vi "Bin WebDav Logging Message Loop.vi"(8 "error in (no error)":errorcluster, 10 "Data Queue":refnum<queue>, 11 "Message Queues":T1) -> (0 "error out":errorcluster)   [LabVIEW 2018, in "Logging.lvlib"]
uses:
  Logging.lvlib
  support/Message Queue/All Message Queues.ctl
  support/Message Queue/Message Cluster.ctl
  Logging Configuration.ctl
  Logging State.ctl
  support/Message Queue/Enqueue Message (Single).vi
  <vilib>/Utility/error.llb/Error Cluster From Error Code.vi
  <vilib>/ErrorRing/Error Ring.xnode
  support/Message Queue/Message Queue.lvlib
  Acquisition/Acquisition.lvlib
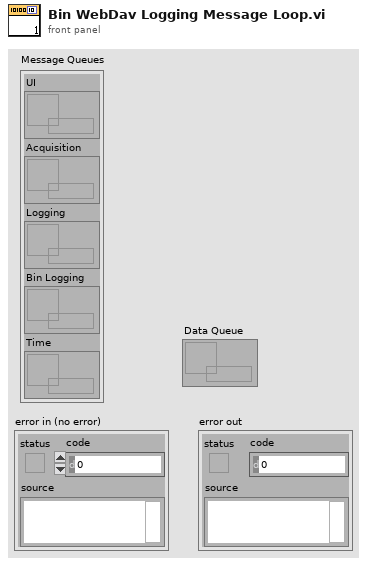
[diagram p1: front panel]
types:
  T1 = typedef "Message Queue.lvlib/All Message Queues.ctl" = cluster{"UI":refnum<queue>, "Acquisition":refnum<queue>, "Logging":refnum<queue>, "Bin Logging":refnum<queue>, "Time":refnum<queue>}
  T2 = typedef "Logging.lvlib/Logging Configuration.ctl" = cluster{"Log File Base Path":path, "TDMS File Reference":refnum<k34>, "Log File Offsite Path":path, "Project code":string, "Bin File Reference":refnum<k34>}
  T3 = typedef "Logging.lvlib/Logging State.ctl" = enum16{"Idle", "Logging"}
  T4 = enum16{"open", "open or create", "create or replace", "create", "open (read-only)"}
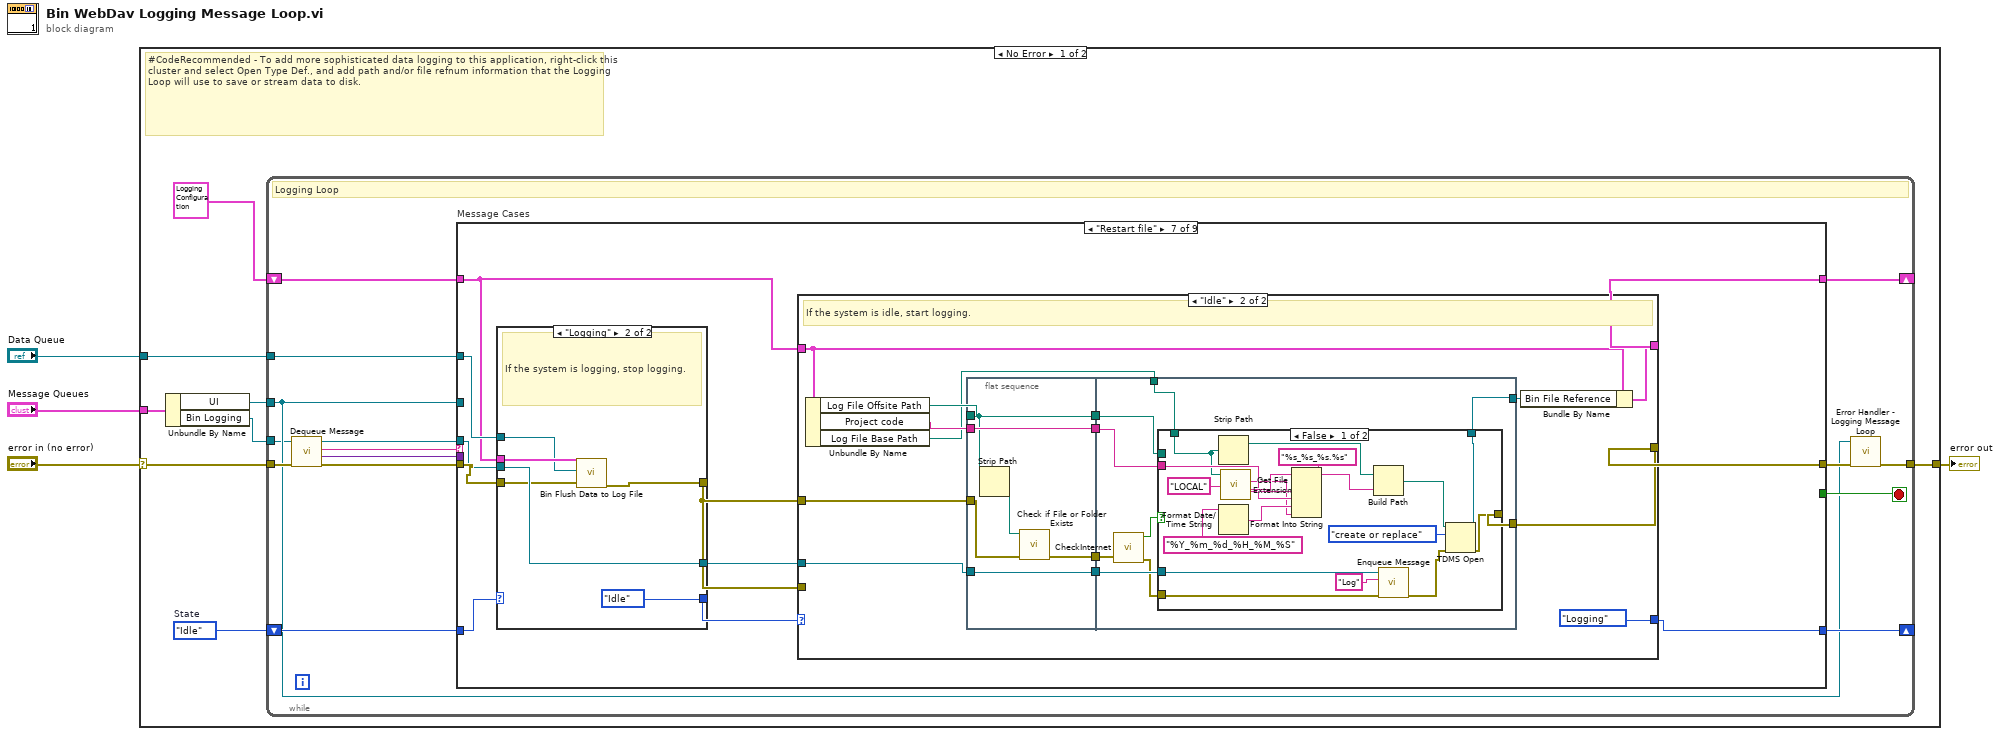
[diagram p0: block diagram]
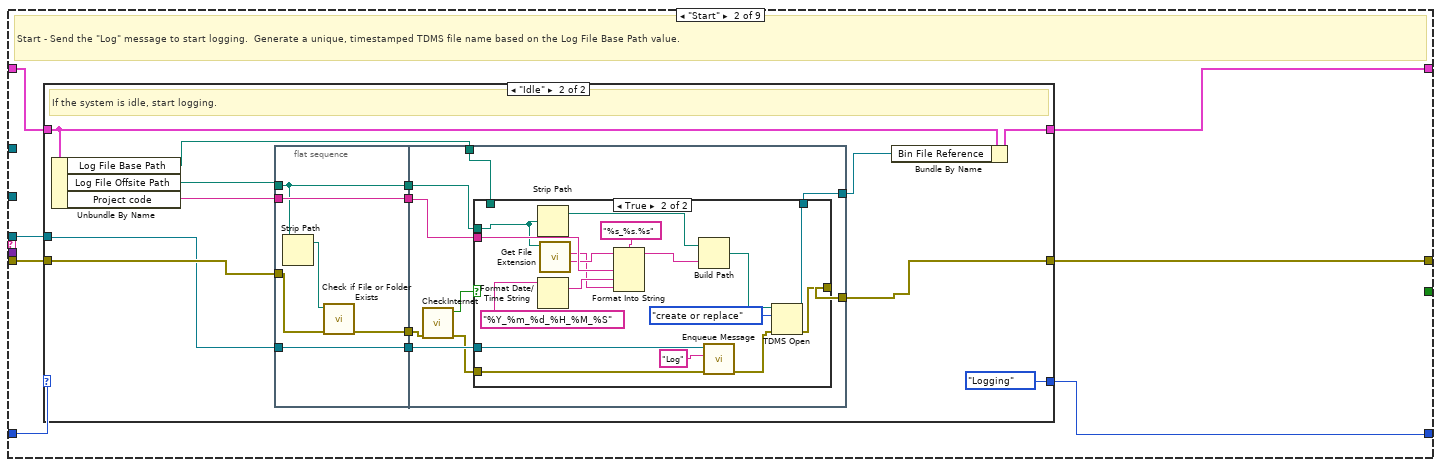
[diagram p3: hidden frame]
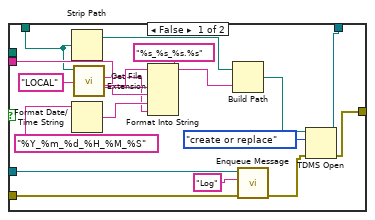
[diagram p5: hidden frame]
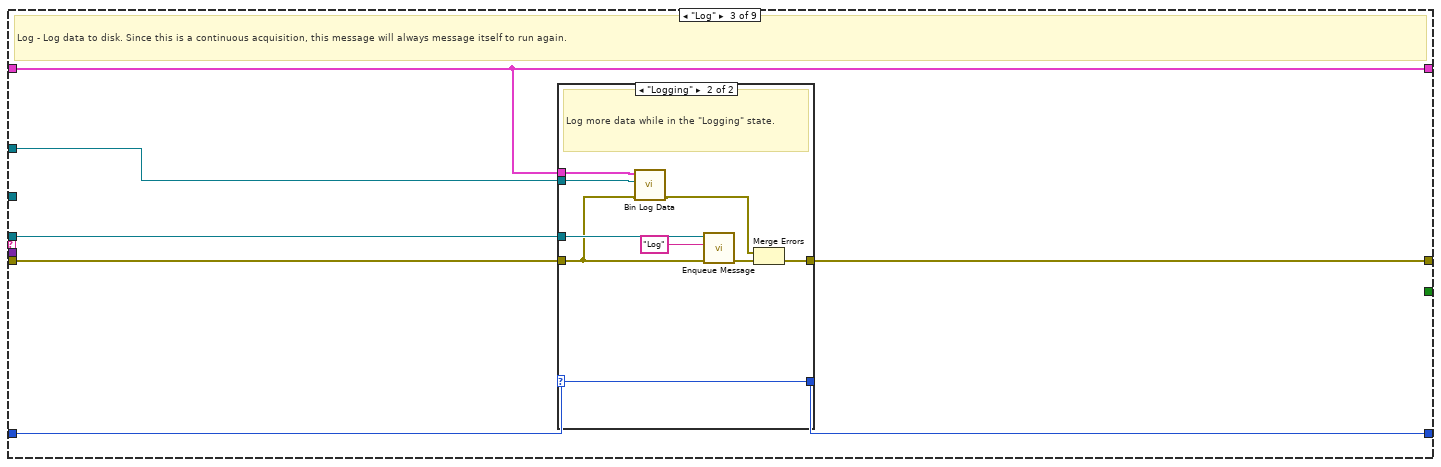
[diagram p6: hidden frame]
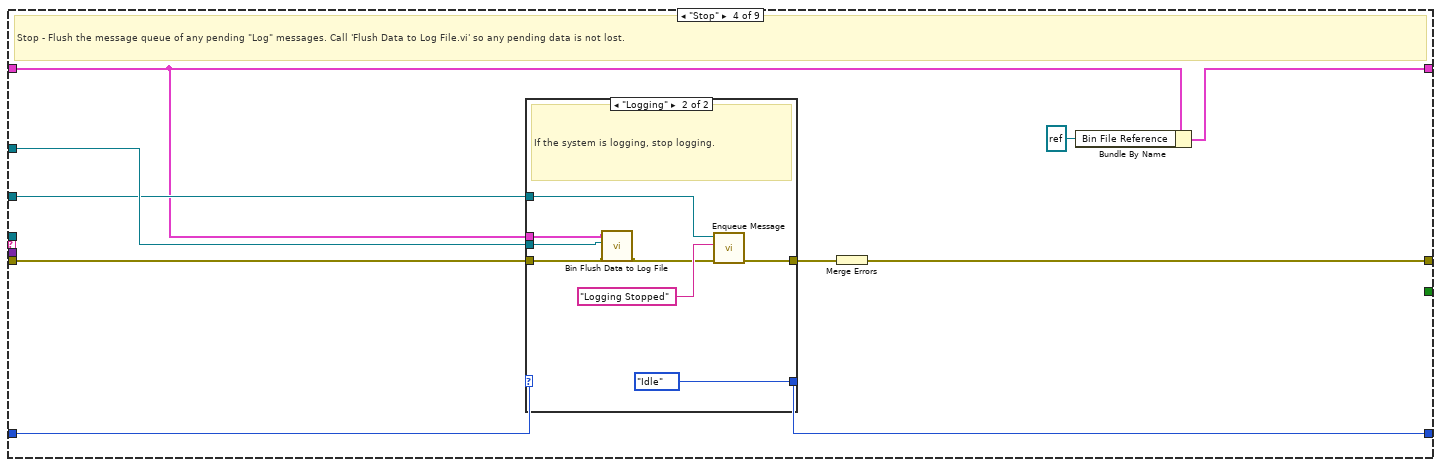
[diagram p8: hidden frame]
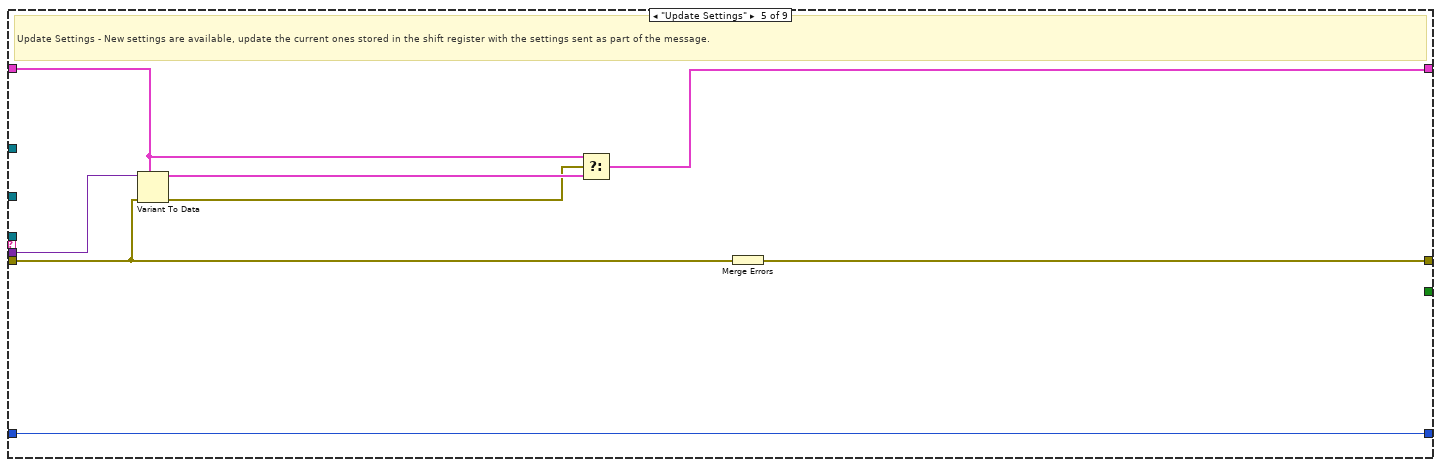
[diagram p10: hidden frame]
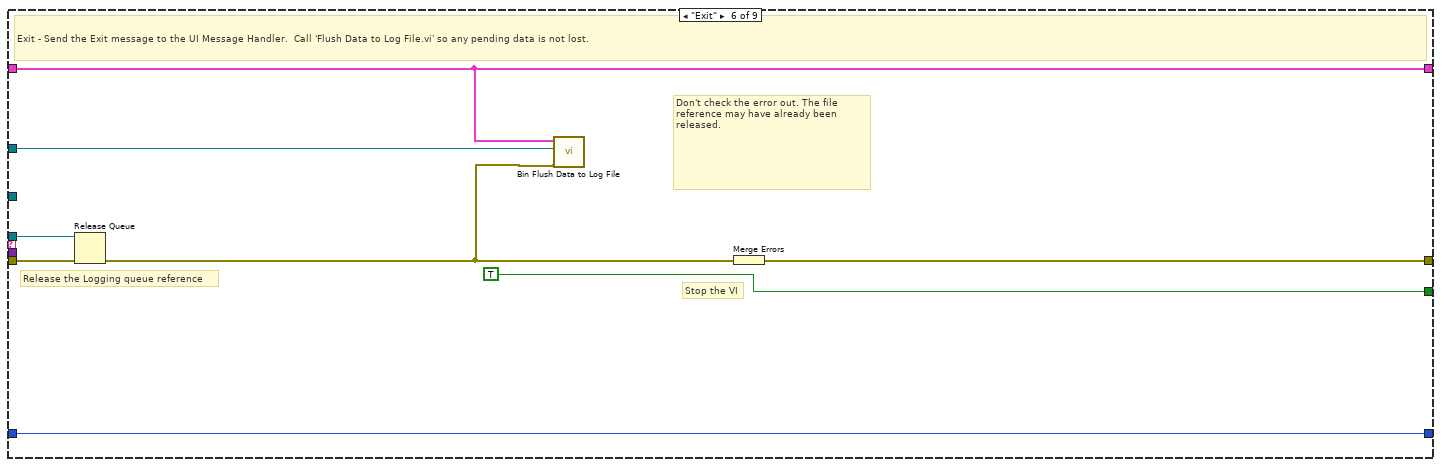
[diagram p11: hidden frame]
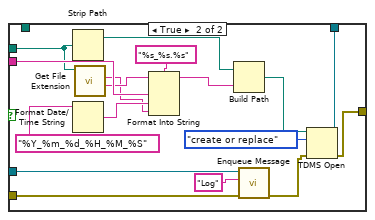
[diagram p13: hidden frame]
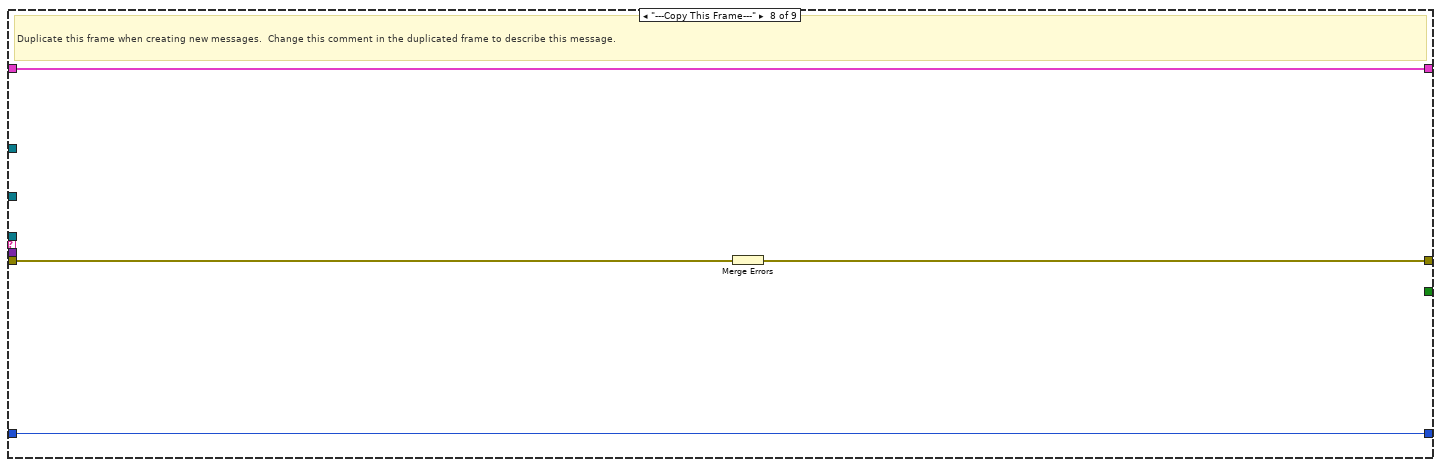
[diagram p15: hidden frame]
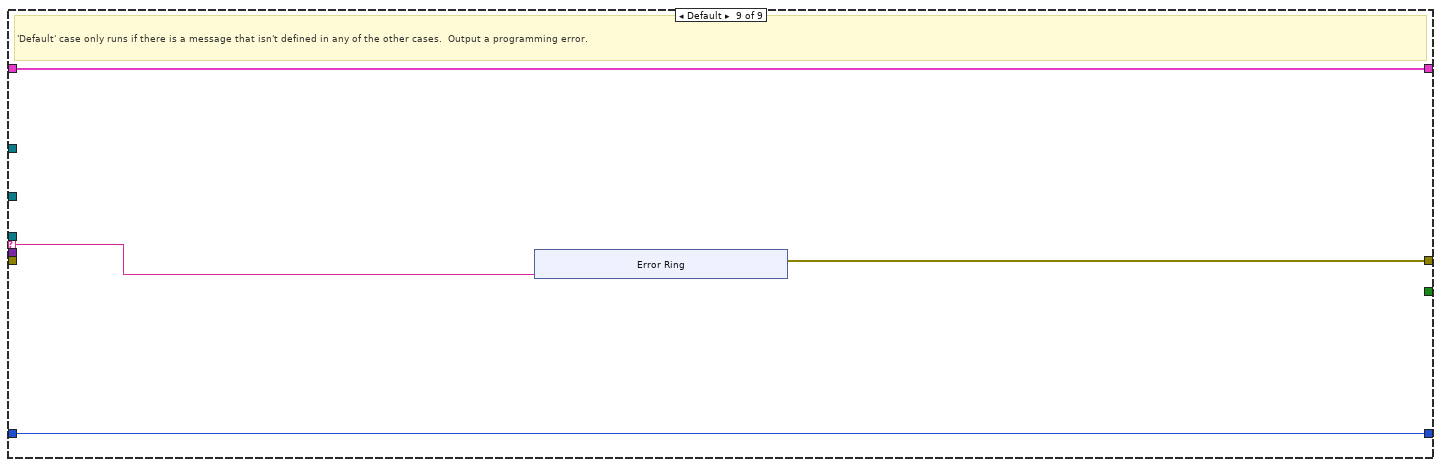
[diagram p16: hidden frame]
diagram:
  n1 = case shown="No Error" "error in (no error)" {
    selector: "error in (no error)" -> [w9 w256]
    tunnel: "Message Queues" -> [w12 _]
    tunnel: [w11 w256] -> w3
    tunnel: "Data Queue" -> [w8 _]
    frame No Error {
      w6 = Logging_State."Idle"  # State
      # "#CodeRecommended - To add more sophisticated data logging to this application, right-click this cluster and select Open Type Def., and add path and/or file refnum information that the Logging Loop will use to save or stream data to disk."
      n2 = Unbundle By Name(w12) -> ("UI"=w7:refnum<queue>, "Bin Logging"=w5:refnum<queue>)
      n3 = while {
        shift-right: [w27] -> _
        shift-left: T2 {"Log File Base Path"=path "", "TDMS File Reference"=refnum, "Log File Offsite Path"=path "", "Project code"="", "Bin File Reference"=refnum} ("Logging Configuration") -> [w14]
        tunnel: w7 -> [w16]
        tunnel: w8 -> [w21]
        shift-right: [w19] -> _
        shift-left: w6 -> [w20]
        tunnel: w9 -> [w25]
        tunnel: [w18] -> w11
        tunnel: w5 -> [w15]
        stop <- w26 stop-if-true
        # "Logging Loop"
        n4 = call "Dequeue Message.vi"("error in (no error)"=w25, "Message Queue"=w15) -> ("error out"=w24:errorcluster, "Message Data"=w23:variant, "Message"=w13:string, "dup Message Queue"=w22:refnum<queue>)  [unwired: 6 in]
        n5 = case "Message Cases" shown="\"Restart file\"" w13 {
          selector: w13 -> [_ _ _ _ _ _ _ _ w245]
          tunnel: w22 -> [_ w36 w108 _ _ w153 w166 _ _]
          tunnel: w24 -> [w29 w35 w106 w127 w141 w154 w167 w244 _]
          tunnel: [w29 w37 w109 w130 w148 w155 w165 w242 w246] -> w17
          tunnel: w14 -> [w30 w34 w105 w123 w147 w151 w161 w243 w248]
          tunnel: [w30 w33 w105 w122 w144 w151 w164 w243 w248] -> w27
          tunnel: [_ _ _ _ _ TRUE _ _ _] -> w26
          tunnel: w23 -> [_ _ _ _ w142 _ _ _ _]
          tunnel: w16 -> [_ _ _ w124 _ _ _ _ _]
          tunnel: w21 -> [_ _ w107 w128 _ w150 w162 _ _]
          tunnel: w20 -> [w28 w32 w104 w126 w143 w152 w163 w241 w247]
          tunnel: [w28 w31 w103 w125 w143 w152 w159 w241 w247] -> w19
          frame "Initialize" {
            # "Initialize - gets called when first launched. Currently a no-op."
          }
          frame "Start" {
            # "Start - Send the \"Log\" message to start logging.  Generate a unique, timestamped TDMS file name based on the Log File Base Path value."
            n6 = case shown="\"Idle\"" w32 {
              selector: w32 -> [w39 _]
              tunnel: [w38 w44] -> w37
              tunnel: w36 -> [_ w45]
              tunnel: w35 -> [w38 w47]
              tunnel: w34 -> [w40 w52]
              tunnel: [w40 w54] -> w33
              tunnel: [w39 Logging_State."Logging" ("State")] -> w31
              frame "Logging" {
                # "The system is already logging. Ignore the \"Start\" message."
              }
              frame "Idle" {
                # "If the system is idle, start logging."
                n7 = Unbundle By Name(w52) -> ("Log File Base Path"=w42:path, "Log File Offsite Path"=w43:path, "Project code"=w46:string)
                n8 = flat-sequence {
                  tunnel: w45 -> [w59]
                  tunnel: w43 -> [w56]
                  tunnel: w46 -> [w60]
                  tunnel: [w57] -> w51
                  tunnel: [w60] -> w50
                  tunnel: [w56] -> w49
                  tunnel: [w59] -> w48
                  tunnel: w47 -> [w58]
                  tunnel: [w69] -> w44
                  tunnel: w51 -> [w64]
                  tunnel: w50 -> [w68]
                  tunnel: w49 -> [w66]
                  tunnel: w48 -> [w67]
                  tunnel: w42 -> [w65]
                  tunnel: [w61] -> w41
                  frame #0 {
                    n9 = Strip Path(path=w56) -> (stripped path=w55:path)  [unwired: 1 out]
                    n10 = call <vilib>:"Check if File or Folder Exists.vi"("error in (no error)"=w58, "path"=w55) -> ("error out"=w57:errorcluster)  [unwired: 7 in, 2 out]
                  }
                  frame #1 {
                    n11 = call "CheckInternet.vi"("error in (no error)"=w64) -> ("error out"=w63:errorcluster, "Available"=w62:bool)  [unwired: 8 in, 1 out]
                    n12 = case shown="True" w62 {
                      tunnel: [w71 w89] -> w69
                      tunnel: w63 -> [w74 w102]
                      tunnel: w68 -> [w78 w101]
                      tunnel: w67 -> [w75 w100]
                      tunnel: w66 -> [_ w91]
                      tunnel: w65 -> [w73 _]
                      tunnel: [w72 w88] -> w61
                      frame False {
                        n13 = Strip Path(path=w73) -> (stripped path=w84:path)  [unwired: 1 out]
                        n14 = Format Date/Time String(time format string (%c)="%Y_%m_%d_%H_%M_%S") -> (date/time string=w82:string)  [unwired: 2 in]
                        n15 = call <vilib>:"Get File Extension.vi"("file"=w73) -> ("filename without extension"=w85:string, "lowercase file extension"=w70:string)  [unwired: 6 in, 3 out]
                        n16 = Format Into String(format string="%s_%s_%s.%s", initial string=w85, "LOCAL" ("input 1"), w78, w82, w70) -> (resulting string=w81:string)  [unwired: 1 in, 1 out]
                        n17 = Build Path(base path=w84, name or relative path=w81) -> (appended path=w80:path)
                        n18 = call-poly "Enqueue Message.vi"("error in (no error)"=w74, "Message"="Log", "Message Queue"=w75) -> ()  [unwired: 7 in, 2 out]
                        n19 = TDMS Open(8:w74, 10:T4."create or replace" ("operation (0:open)"), 11:w80) -> (0:w71:errorcluster, 3:w72:refnum<k34>)  [unwired: 4 in]
                      }
                      frame True {
                        n20 = Strip Path(path=w91) -> (stripped path=w96:path)  [unwired: 1 out]
                        n21 = Format Date/Time String(time format string (%c)="%Y_%m_%d_%H_%M_%S") -> (date/time string=w94:string)  [unwired: 2 in]
                        n22 = call <vilib>:"Get File Extension.vi"("file"=w91) -> ("filename without extension"=w97:string, "lowercase file extension"=w87:string)  [unwired: 6 in, 3 out]
                        n23 = Format Into String(format string="%s_%s.%s", initial string=w97, w101, w94, w87) -> (resulting string=w93:string)  [unwired: 1 in, 1 out]
                        n24 = Build Path(base path=w96, name or relative path=w93) -> (appended path=w92:path)
                        n25 = call-poly "Enqueue Message.vi"("error in (no error)"=w102, "Message"="Log", "Message Queue"=w100) -> ()  [unwired: 7 in, 2 out]
                        n26 = TDMS Open(8:w102, 10:T4."create or replace" ("operation (0:open)"), 11:w92) -> (0:w89:errorcluster, 3:w88:refnum<k34>)  [unwired: 4 in]
                      }
                    }
                  }
                }
                n27 = Bundle By Name(cluster=w52, "Bin File Reference"=w41) -> (w54:T2)
              }
            }
          }
          frame "Log" {
            # "Log - Log data to disk. Since this is a continuous acquisition, this message will always message itself to run again."
            n28 = case shown="\"Logging\"" w104 {
              selector: w104 -> [w111 w116]
              tunnel: [w110 w120] -> w109
              tunnel: w108 -> [_ w118]
              tunnel: w107 -> [_ w114]
              tunnel: w106 -> [w110 w113]
              tunnel: w105 -> [_ w115]
              tunnel: [w111 w116] -> w103
              frame "Idle" {
                # "Ignore \"Log\" messages when the logging is idle."
              }
              frame "Logging" {
                # "Log more data while in the \"Logging\" state."
                n29 = call "Bin Log Data.vi"("error in (no error)"=w113, "Data Queue"=w114, "Logging Configuration"=w115) -> ("error out"=w112:errorcluster)  [unwired: 8 in]
                n30 = call-poly "Enqueue Message.vi"("error in (no error)"=w113, "Message"="Log", "Message Queue"=w118) -> ("error out"=w119:errorcluster)  [unwired: 7 in, 1 out]
                n31 = Merge Errors(w112, w119) -> (w120:errorcluster)
              }
            }
          }
          frame "Stop" {
            # "Stop - Flush the message queue of any pending \"Log\" messages. Call 'Flush Data to Log File.vi' so any pending data is not lost."
            n32 = case shown="\"Logging\"" w126 {
              selector: w126 -> [w131 _]
              tunnel: [w132 w133] -> w129
              tunnel: w128 -> [_ w136]
              tunnel: w123 -> [_ w137]
              tunnel: w127 -> [w132 w135]
              tunnel: [w131 Logging_State."Idle" ("State")] -> w125
              tunnel: w124 -> [_ w139]
              frame "Idle" {
                # "The system is already idle. Ignore the \"Stop\" message."
              }
              frame "Logging" {
                # "If the system is logging, stop logging."
                n33 = call "Bin Flush Data to Log File.vi"("error in (no error)"=w135, "Data Queue"=w136, "Logging Configuration"=w137) -> ("error out"=w134:errorcluster)  [unwired: 8 in]
                n34 = call-poly "Enqueue Message.vi"("error in (no error)"=w134, "Message"="Logging Stopped", "Message Queue"=w139) -> ("error out"=w133:errorcluster)  [unwired: 7 in, 1 out]
              }
            }
            n35 = Merge Errors(w129) -> (w130:errorcluster)
            n36 = Bundle By Name(cluster=w123, "Bin File Reference"=refnum<k34> refnum) -> (w122:T2)
          }
          frame "Update Settings" {
            # "Update Settings - New settings are available, update the current ones stored in the shift register with the settings sent as part of the message."
            n37 = Variant To Data(error in=w141, type=w147, Variant=w142) -> (data=w146:T2, error out=w145:errorcluster)
            n38 = Select(t=w147, s=w145, f=w146) -> (s? t:f=w144:T2)
            n39 = Merge Errors(w141) -> (w148:errorcluster)
          }
          frame "Exit" {
            # "Don't check the error out. The file reference may have already been released."
            # "Release the Logging queue reference"
            # "Stop the VI"
            # "Exit - Send the Exit message to the UI Message Handler.  Call 'Flush Data to Log File.vi' so any pending data is not lost."
            n40 = Release Queue(queue=w153, error in (no error)=w154) -> (error out=w149:errorcluster)  [unwired: 1 in, 2 out]
            n41 = call "Bin Flush Data to Log File.vi"("error in (no error)"=w149, "Data Queue"=w150, "Logging Configuration"=w151) -> ()  [unwired: 8 in, 1 out]
            n42 = Merge Errors(w149) -> (w155:errorcluster)
          }
          frame "Restart file" {
            n43 = case shown="\"Logging\"" w163 {
              selector: w163 -> [w233 _]
              tunnel: [w234 w235] -> w158
              tunnel: w166 -> [_ w239]
              tunnel: w161 -> [_ w238]
              tunnel: w167 -> [w234 w236]
              tunnel: [w233 Logging_State."Idle" ("State")] -> w160
              tunnel: w162 -> [_ w237]
              tunnel: [_ w239] -> w157
              frame "Idle" {
                # "The system is already idle. Ignore the \"Stop\" message."
              }
              frame "Logging" {
                # "If the system is logging, stop logging."
                n44 = call "Bin Flush Data to Log File.vi"("error in (no error)"=w236, "Data Queue"=w237, "Logging Configuration"=w238) -> ("error out"=w235:errorcluster)  [unwired: 8 in]
              }
            }
            n45 = case shown="\"Idle\"" w160 {
              selector: w160 -> [w170 _]
              tunnel: [w169 w183] -> w165
              tunnel: [w168 w178] -> w164
              tunnel: [w170 Logging_State."Logging" ("State")] -> w159
              tunnel: w161 -> [w168 w179]
              tunnel: w158 -> [w169 _]
              tunnel: w157 -> [_ w180]
              tunnel: w158 -> [_ w173]
              frame "Logging" {
                # "The system is already logging. Ignore the \"Start\" message."
              }
              frame "Idle" {
                # "If the system is idle, start logging."
                n46 = Unbundle By Name(w179) -> ("Log File Offsite Path"=w181:path, "Project code"=w182:string, "Log File Base Path"=w172:path)
                n47 = flat-sequence {
                  tunnel: w180 -> [w189]
                  tunnel: w181 -> [w186]
                  tunnel: w182 -> [w190]
                  tunnel: [w187] -> w177
                  tunnel: [w190] -> w176
                  tunnel: [w186] -> w175
                  tunnel: [w189] -> w174
                  tunnel: w173 -> [w188]
                  tunnel: [w199] -> w183
                  tunnel: [w196] -> w171
                  tunnel: w177 -> [w193]
                  tunnel: w176 -> [w198]
                  tunnel: w175 -> [w195]
                  tunnel: w174 -> [w197]
                  tunnel: w172 -> [w194]
                  frame #0 {
                    n48 = Strip Path(path=w186) -> (stripped path=w185:path)  [unwired: 1 out]
                    n49 = call <vilib>:"Check if File or Folder Exists.vi"("error in (no error)"=w188, "path"=w185) -> ("error out"=w187:errorcluster)  [unwired: 7 in, 2 out]
                  }
                  frame #1 {
                    n50 = call "CheckInternet.vi"("error in (no error)"=w193) -> ("error out"=w192:errorcluster, "Available"=w191:bool)  [unwired: 8 in, 1 out]
                    n51 = case shown="False" w191 {
                      tunnel: [w202 w220] -> w199
                      tunnel: w192 -> [w205 w232]
                      tunnel: w198 -> [w209 w231]
                      tunnel: w197 -> [w206 w230]
                      tunnel: [w203 w218] -> w196
                      tunnel: w195 -> [_ w221]
                      tunnel: w194 -> [w204 _]
                      frame False {
                        n52 = Strip Path(path=w204) -> (stripped path=w214:path)  [unwired: 1 out]
                        n53 = Format Date/Time String(time format string (%c)="%Y_%m_%d_%H_%M_%S") -> (date/time string=w212:string)  [unwired: 2 in]
                        n54 = call <vilib>:"Get File Extension.vi"("file"=w204) -> ("filename without extension"=w215:string, "lowercase file extension"=w200:string)  [unwired: 6 in, 3 out]
                        n55 = Format Into String(format string="%s_%s_%s.%s", initial string=w215, "LOCAL" ("input 1"), w209, w212, w200) -> (resulting string=w211:string)  [unwired: 1 in, 1 out]
                        n56 = Build Path(base path=w214, name or relative path=w211) -> (appended path=w210:path)
                        n57 = call-poly "Enqueue Message.vi"("error in (no error)"=w205, "Message"="Log", "Message Queue"=w206) -> ()  [unwired: 7 in, 2 out]
                        n58 = TDMS Open(8:w205, 10:T4."create or replace" ("operation (0:open)"), 11:w210) -> (0:w202:errorcluster, 3:w203:refnum<k34>)  [unwired: 4 in]
                      }
                      frame True {
                        n59 = Strip Path(path=w221) -> (stripped path=w226:path)  [unwired: 1 out]
                        n60 = Format Date/Time String(time format string (%c)="%Y_%m_%d_%H_%M_%S") -> (date/time string=w224:string)  [unwired: 2 in]
                        n61 = call <vilib>:"Get File Extension.vi"("file"=w221) -> ("filename without extension"=w227:string, "lowercase file extension"=w217:string)  [unwired: 6 in, 3 out]
                        n62 = Format Into String(format string="%s_%s.%s", initial string=w227, w231, w224, w217) -> (resulting string=w223:string)  [unwired: 1 in, 1 out]
                        n63 = Build Path(base path=w226, name or relative path=w223) -> (appended path=w222:path)
                        n64 = call-poly "Enqueue Message.vi"("error in (no error)"=w232, "Message"="Log", "Message Queue"=w230) -> ()  [unwired: 7 in, 2 out]
                        n65 = TDMS Open(8:w232, 10:T4."create or replace" ("operation (0:open)"), 11:w222) -> (0:w220:errorcluster, 3:w218:refnum<k34>)  [unwired: 4 in]
                      }
                    }
                  }
                }
                n66 = Bundle By Name(cluster=w179, "Bin File Reference"=w171) -> (w178:T2)
              }
            }
          }
          frame "---Copy This Frame---" {
            # "Duplicate this frame when creating new messages.  Change this comment in the duplicated frame to describe this message."
            n67 = Merge Errors(w244) -> (w242:errorcluster)
          }
          frame Default {
            # "'Default' case only runs if there is a message that isn't defined in any of the other cases.  Output a programming error."
            n68 = xnode "Error Ring"("parameter 0"=w245) -> ("error out"=w246:errorcluster)
          }
        }
        n69 = call "Error Handler - Logging Message Loop.vi"("error in (no error)"=w17, "Message Queue"=w16) -> ("dup error in"=w18:errorcluster)  [unwired: 8 in, 1 out]
      }
    }
    frame Error {
    }
  }
  "error out" <- w3
